vi "rs232_qsm.vi"   [LabVIEW 2013]
uses:
  labview/power_vi_stm_v13_1_7_22/labview/gen_libs/non_instr/gen_ctls/enums/state_enum.ctl
  labview/power_vi_stm_v13_1_7_22/labview/gen_libs/non_instr/gen_ctls/gen_ctls/ue_ref_clstr.ctl
  labview/power_vi_stm_v13_1_7_22/labview/gen_libs/instr/instr_ctls/instr_usr_evnt_clstr.ctl
  labview/power_vi_stm_v13_1_7_22/labview/gen_libs/instr/instr_ctls/res_tsk_out_clstr.ctl
  labview/power_vi_stm_v13_1_7_22/labview/gen_libs/instr/instr_ctls/keys_e36313a_params.ctl
  labview/power_vi_stm_v13_1_7_22/labview/projects/shell_to_shell/main_shell_to_shell_clstr.ctl
  labview/power_vi_stm_v13_1_7_22/labview/gen_libs/instr/instr_ctls/data_qtp_1133_clstr.ctl
  labview/power_vi_stm_v13_1_7_22/labview/gen_libs/instr/instr_ctls/ni_9205_params.ctl
  labview/power_vi_stm_v13_1_7_22/labview/gen_libs/instr/instr_ctls/ni_9213_params.ctl
  labview/power_vi_stm_v13_1_7_22/labview/gen_libs/instr/instr_ctls/ni_9205_volt_cal_params.ctl
  labview/power_vi_stm_v13_1_7_22/labview/gen_libs/both/gen_ctls/main_clstr.ctl
  labview/power_vi_stm_v13_1_7_22/labview/gen_libs/instr/instr_ctls/ni_8731a_params.ctl
  labview/power_vi_stm_v13_1_7_22/labview/gen_libs/non_instr/gen_ctls/gen_ctls/pwr_vi_test.ctl
  labview/power_vi_stm_v13_1_7_22/labview/gen_libs/instr/instr_ctls/ni_8731a_arry.ctl
  labview/power_vi_stm_v13_1_7_22/labview/gen_libs/instr/instr_ctls/dat_clstr_arry.ctl
  labview/power_vi_stm_v13_1_7_22/labview/gen_libs/instr/instr_ctls/watlow_std_bus.ctl
  labview/power_vi_stm_v13_1_7_22/labview/gen_libs/instr/instr_ctls/oven_settings.ctl
  labview/power_vi_stm_v13_1_7_22/labview/gen_libs/non_instr/gen_ctls/gen_ctls/gen_temp_cyc_clstr.ctl
  labview/power_vi_stm_v13_1_7_22/labview/gen_libs/instr/instr_ctls/daq_type_enum.ctl
  labview/power_vi_stm_v13_1_7_22/labview/gen_libs/instr/instr_ctls/source_type.ctl
  labview/power_vi_stm_v13_1_7_22/labview/gen_libs/instr/instr_ctls/daq_temp_enum.ctl
  labview/power_vi_stm_v13_1_7_22/labview/gen_libs/instr/instr_ctls/data_filtr_type_enum.ctl
  labview/power_vi_stm_v13_1_7_22/labview/gen_libs/instr/instr_ctls/when_to_soak_enum.ctl
  labview/power_vi_stm_v13_1_7_22/labview/gen_libs/instr/instr_ctls/tcp_rem_mon_enum.ctl
  labview/power_vi_stm_v13_1_7_22/labview/gen_libs/non_instr/gen_ctls/enums/temp_cond_enum.ctl
  labview/power_vi_stm_v13_1_7_22/labview/gen_libs/both/gen_ctls/rs232_data_clstr.ctl
  event_clstr.ctl
  states_cntrl.ctl
  log_dat.ctl
  temp_ind.ctl
  rh_ind_arry.ctl
  rh_ind.ctl
  sens_type.ctl
  sens_type_arry_cntrl.ctl
  pibs_clstr.ctl
  sens_type_arry_str_cntrl.ctl
  raw_dat_str.ctl
  dts_cntrl.ctl
types:
  T1 = typedef "rs232_data_clstr.ctl" = cluster{"state":T2, "connection ID":refnum<k5>, "stop_evnt_loop":bool, "main_q":refnum<queue>, "bytes read":u32, "Response":string, "wr_buffr":string, "bytes_at_port":u32, "visa_rsc_out":refnum<visa-resource-name>, "delay":u32, "sens_type_arry":T3, "chk_bytes_rd":u32}
  T2 = typedef "state_enum.ctl" = enum16{"idle", "exit", "obtain_q", "init", "create_file", "pik_sampl_mode", "init_instr_finite", "init_instr_cont", "update_file_path", "change_v_setting", "change _i_range", "turn_on_cur_qry", "turn_on_tst_cur", "dwell", "temp_stb_dwell", "meas", "v_set_qry", "range_qry", "save_data", "display_data", "cmd_proxy_state", "setting_proxy_state", "turn_off_tst_cur", "turn_off_curr_to_stop", "max_turn_off_trials_qry", "exit_prog", "max_trials_qry", "empty_str_qry", "man_cmd_qry", "man_cmd_qry_after_x_times", "cyc_qry", "turn_on_tcm", "turn_off_tcm", "chk_for_tcm", "max_trials_for_tcm", "turn_on_init_tcm", "srch_for_all_files", "strt_pdf_file", "append_pic", "append_header", "append_new_page", "pics_done_qry", "close_pdf_file", "set_cal_volt", "meas_cal_volt", "incr_voltage", "incr_cur_g1", "incr_cur_g2", "first_last_cyc_qry", "compare_results", "update_params", "cont_meas", "set_first_cur", "test_done_qry", "init_m3_temp_qry", "m3_diff_temp_qry", "temp_rched_qry", "set_init_oven_temp", "oven_temp_dwell", "update_oven_settings", "meas_oven_temp", "oven_temp_diff", "get_dat_from_vis", "ret_dat_from_cdaq", "ret_dat_from_ps", "close_cont_daqs", "cyc_trig_qry", "hot_temp_trig_qry", "cold_temp_trig_qry", "amb_temp_trig_qry", "both_temps_trig_qry", "temp_cond_hot_qry", "temp_cond_cold_qry", "temp_cond_amb_qry", "dur_strt_qry", "dur_end_qry", "daq_per_trig_qry", "src_type_qry", "turn_on_ps_1", "turn_off_ps_1", "turn_on_ps_2", "turn_off_ps_2", "data_type_qry", "user_stop_qry", "ret_data", "stm_snd_to_client", "strt_stm_listen", "snd_cmd", "capt_wait", "read_data", "chk_bytes_rd"}
  T3 = typedef "sens_type_arry_cntrl.ctl" = T4[]
  T4 = typedef "sens_type.ctl" = u8
  T5 = typedef "ue_ref_clstr.ctl" = cluster{"instr_usr_evnt_ref":refnum<user-event>, "key_e36313a_params_usr_evnt":refnum<user-event>, "main_stop_ue_ref":refnum<user-event>, "main_shell_to_shell_params":refnum<user-event>, "main_clstr_ref":refnum<user-event>, "stp_evnt_loop":refnum<user-event>}
  T6 = typedef "states_cntrl.ctl" = enum16{"idle", "exit", "init", "obtain_q", "capt_data", "snd_sens_type", "send_cmd", "capt_wait", "read_data", "chk_bytes_rd", "disp_data", "sav_qry", "sav_dat", "dwell", "small_dwell", "stop_capt_qry", "go_to_minor_qsm", "retr_data", "auto_in_minor_qsm"}
  T7 = typedef "event_clstr.ctl" = cluster{"states":T6, "bytes read":u32, "Response":string, "wr_buffr":string, "bytes_at_port":u32, "temp_clstr":T8, "logTable in":string[][][], "mult_list":i32, "log_tabl_row_cnt":u64, "above_row_7":bool, "sens_type":T4, "sens_type_arry":T3, "pibs_clstr":T12, "dts":T15}
  T8 = typedef "log_dat.ctl" = cluster{"sen_4_num":T9, "sen_3_num":T9, "sen_2_num":T9, "sen_1_num":T9, "sen_8_num":T9, "sen_7_num":T9, "sen_6_num":T9, "sen_5_num":T9, "dts":string, "sen_4":string, "sen_3":string, "sen_2":string, "sen_1":string, "sen_8":string, "sen_7":string, "sen_6":string, "sen_5":string, "temp_f_arry":T9[], "sens_dat_raw_arry":string[], "raw_dat":string, "rh_arry":T10, "rh_1":T11, "rh_0":T11, "rh_3":T11, "rh_2":T11, "rh_5":T11, "rh_4":T11, "rh_7":T11, "rh_6":T11}
  T9 = typedef "temp_ind.ctl" = dbl
  T10 = typedef "rh_ind_arry.ctl" = T11[]
  T11 = typedef "rh_ind.ctl" = dbl
  T12 = typedef "pibs_clstr.ctl" = cluster{"sens_typ_str":T13, "rh_1":T11, "sen_8":T14, "sen_7":T14, "sen_6":T14, "sen_5":T14, "sen_4":T14, "sen_3":T14, "sen_2":T14, "sen_1_num":T9, "sen_1":T14, "rh_2":T11, "rh_3":T11, "sen_2_num":T9, "sen_3_num":T9, "sen_4_num":T9, "rh_4":T11, "sen_5_num":T9, "rh_5":T11, "sen_6_num":T9, "rh_6":T11, "sen_7_num":T9, "rh_7":T11, "sen_8_num":T9, "rh_8":T11, "sens_type_1":T4, "sens_type_2":T4, "sens_type_3":T4, "sens_type_4":T4, "sens_type_5":T4, "sens_type_6":T4, "sens_type_7":T4, "sens_type_8":T4, "sens_typ_str _2":T13}
  T13 = typedef "sens_type_arry_str_cntrl.ctl" = string
  T14 = typedef "raw_dat_str.ctl" = string
  T15 = typedef "dts_cntrl.ctl" = string
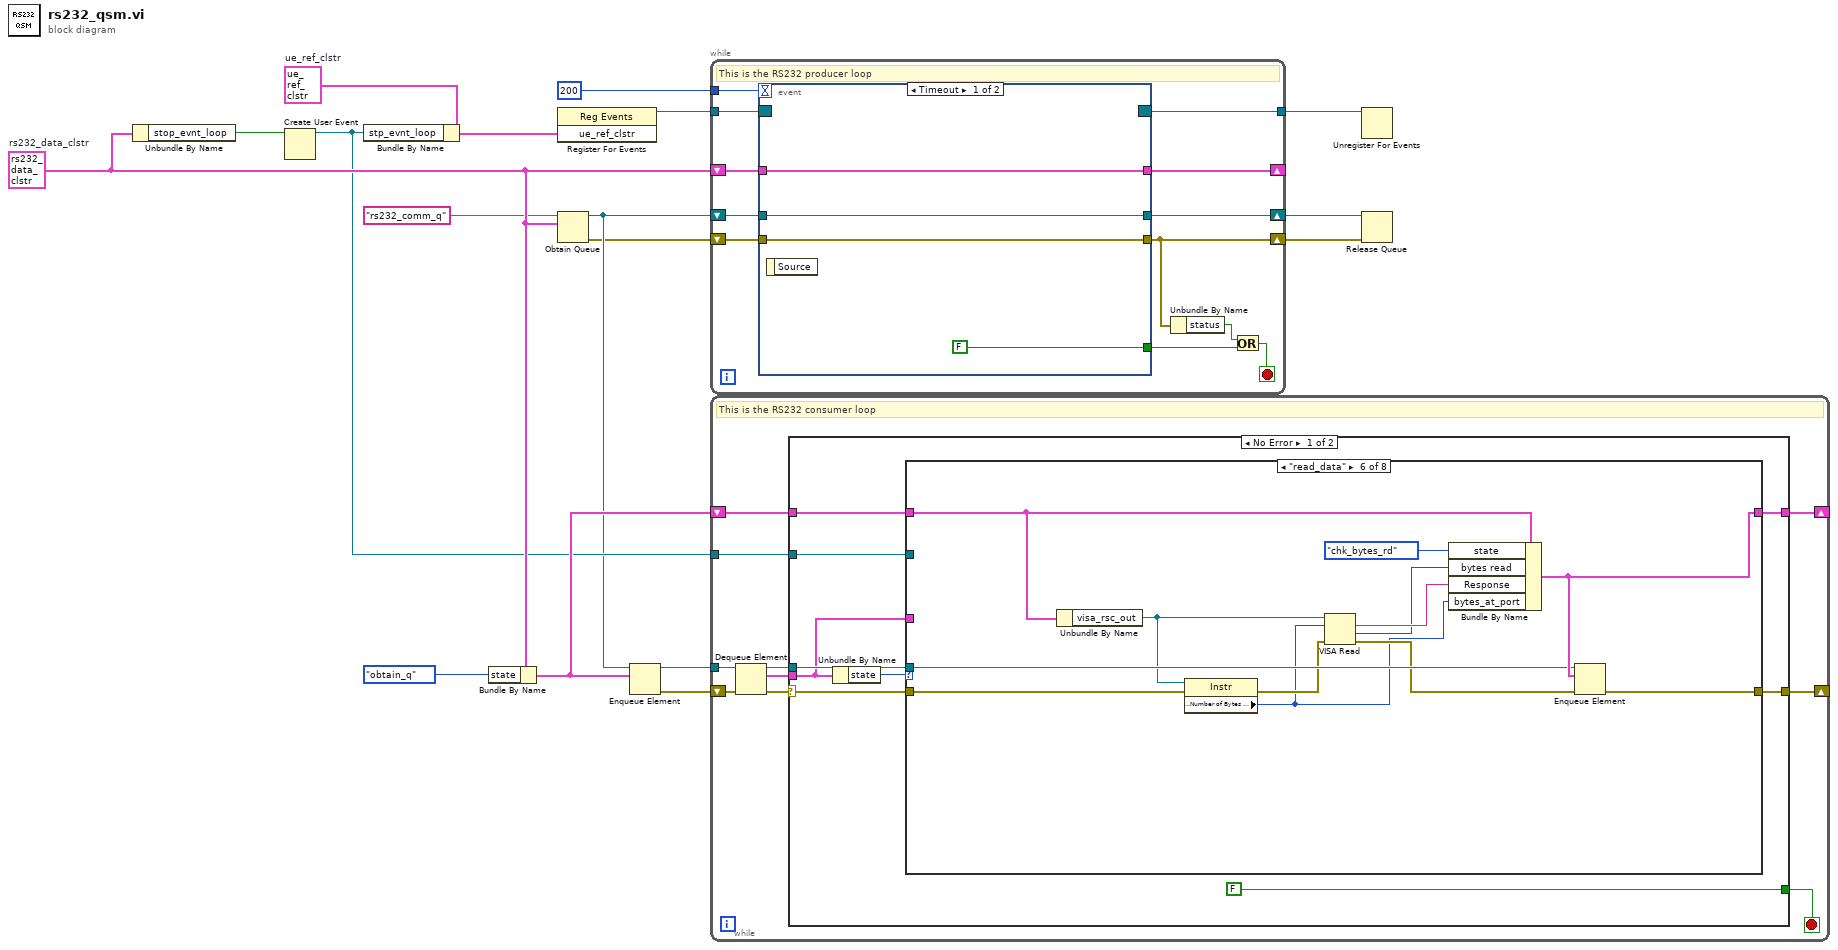
[diagram p0: block diagram]
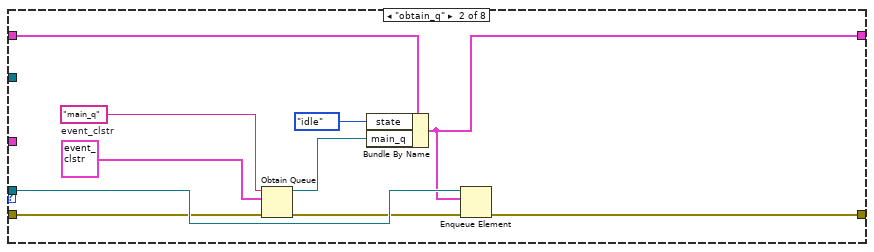
[diagram p3: hidden frame]
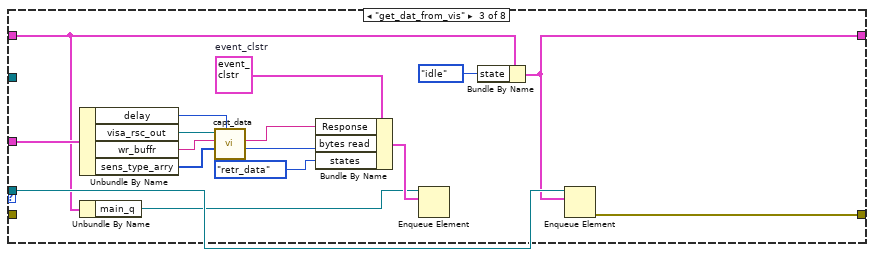
[diagram p4: hidden frame]
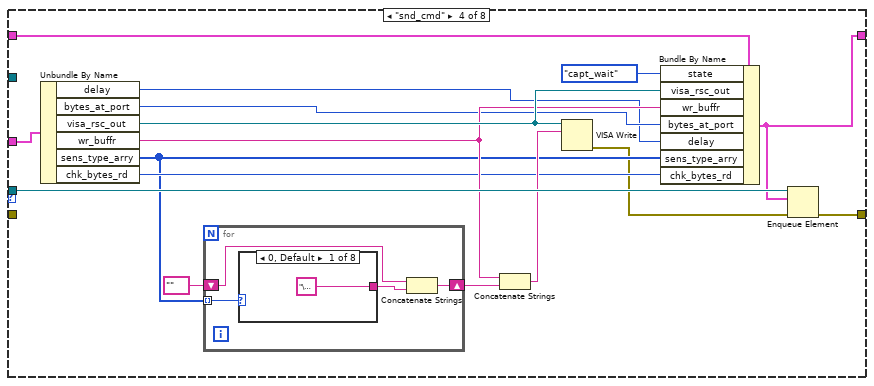
[diagram p5: hidden frame]
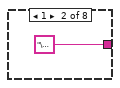
[diagram p6: hidden frame]
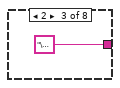
[diagram p7: hidden frame]
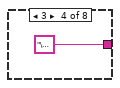
[diagram p8: hidden frame]
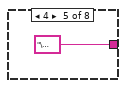
[diagram p9: hidden frame]
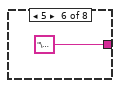
[diagram p10: hidden frame]
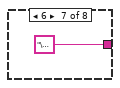
[diagram p11: hidden frame]
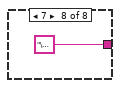
[diagram p12: hidden frame]
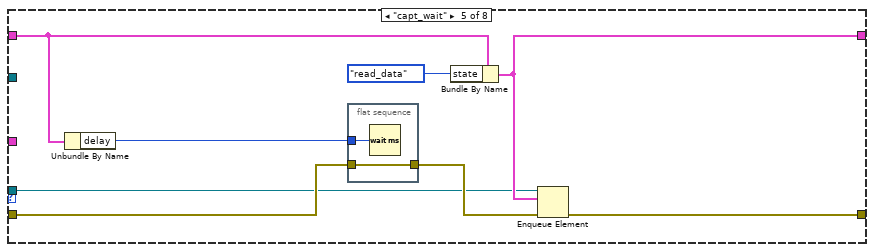
[diagram p13: hidden frame]
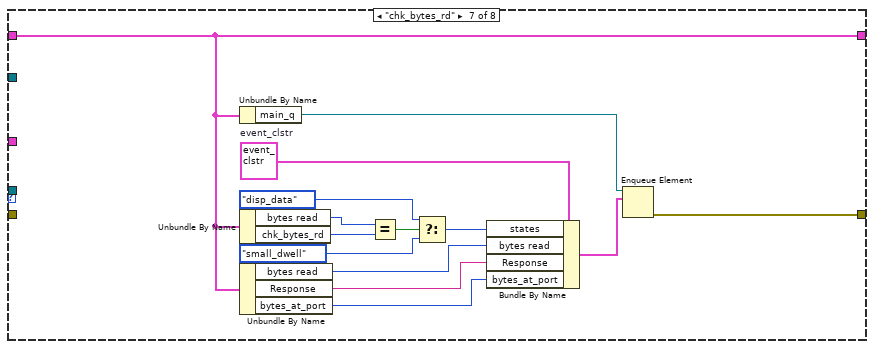
[diagram p14: hidden frame]
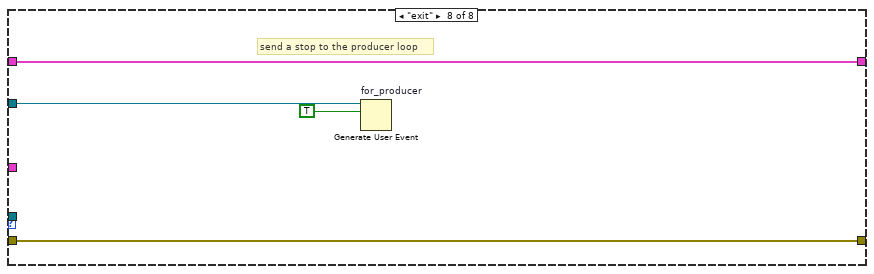
[diagram p15: hidden frame]
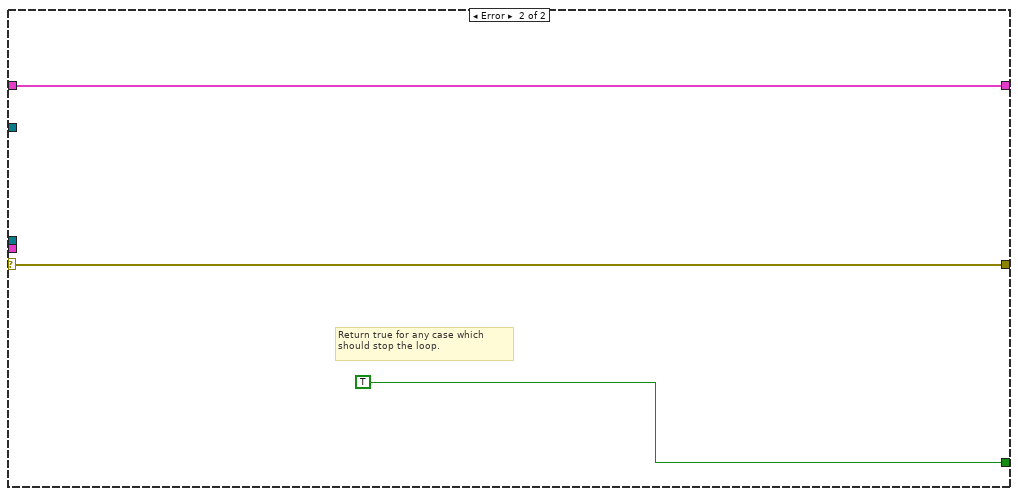
[diagram p16: hidden frame]
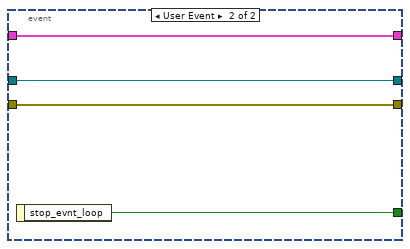
[diagram p17: hidden frame]
diagram:
  w17 = T1 {"state"=enum."idle", "connection ID"=refnum, "stop_evnt_loop"=FALSE, "main_q"=refnum, "bytes read"=0, "Response"="", "wr_buffr"="", "bytes_at_port"=0, "visa_rsc_out"="", "delay"=0, "sens_type_arry"=[], "chk_bytes_rd"=0}  # rs232_data_clstr
  w4 = T5 {"instr_usr_evnt_ref"=refnum, "key_e36313a_params_usr_evnt"=refnum, "main_stop_ue_ref"=refnum, "main_shell_to_shell_params"=refnum, "main_clstr_ref"=refnum, "stp_evnt_loop"=refnum}  # ue_ref_clstr
  n1 = Unbundle By Name(w17) -> ("stop_evnt_loop"=w5:bool)
  n2 = Create User Event(user event datatype=w5) -> (user event=w10:refnum<user-event>)  [unwired: 1 in, 1 out]
  n3 = Bundle By Name(cluster=w4, "stp_evnt_loop"=w10) -> (w3:T5)
  n4 = Bundle By Name(cluster=w17, "state"=state_enum."obtain_q") -> (w12:T1)
  n5 = register-events(w3) -> (reference out=w2:refnum<event-registration>)  [unwired: 2 in, 1 out]
  n6 = Obtain Queue(name (unnamed)="rs232_comm_q", element data type=w17) -> (queue out=w8:refnum<queue>, error out=w7:errorcluster)  [unwired: 3 in, 1 out]
  n7 = Enqueue Element(queue=w8, element=w12) -> (queue out=w9:refnum<queue>, error out=w13:errorcluster)  [unwired: 2 in, 1 out]
  n8 = while {
    shift-right: [w20] -> w16
    shift-left: w7 -> [w27]
    shift-right: [w28] -> w15
    shift-left: w8 -> [w29]
    shift-right: [w24] -> _
    shift-left: w17 -> [w26]
    tunnel: 200 -> [w25]
    tunnel: w2 -> [w23]
    tunnel: [w22] -> w14
    stop <- w18 stop-if-true
    # "This is the RS232 producer loop"
    n9 = event shown="[0] Timeout" {
      selector: w23 -> [_ _]
      dyn-events: [_ _] -> w22
      timeout: w25 -> [_ _]
      tunnel: w29 -> [w32 w36]
      tunnel: [w32 w36] -> w28
      tunnel: w27 -> [w31 w35]
      tunnel: [w31 w35] -> w20
      tunnel: w26 -> [w33 w37]
      tunnel: [w33 w37] -> w24
      tunnel: [FALSE w34] -> w19
      event Timeout {
        n10 = event-data() -> ()  [unwired: 1 in, 1 out]
      }
      event User Event {
        n11 = event-data() -> ("stop_evnt_loop"=w34:bool)  [unwired: 1 in]
      }
    }
    n12 = Unbundle By Name(w20) -> ("status"=w21:bool)
    n13 = Or(x=w21, y=w19) -> (x .or. y?=w18:bool)
  }
  n14 = while {
    tunnel: w9 -> [w47]
    shift-right: [w42] -> _
    shift-left: w12 -> [w43]
    shift-right: [w40] -> _
    shift-left: w13 -> [w44]
    tunnel: w10 -> [w39]
    stop <- w38 stop-if-true
    # "This is the RS232 consumer loop"
    n15 = Dequeue Element(queue=w47, error in (no error)=w44) -> (queue out=w41:refnum<queue>, element=w45:T1, error out=w46:errorcluster)  [unwired: 1 in, 1 out]
    n16 = case shown="No Error" w46 {
      selector: w46 -> [w55 w153]
      tunnel: w45 -> [w49 _]
      tunnel: [FALSE TRUE] -> w38
      tunnel: w43 -> [w54 w154]
      tunnel: [w48 w154] -> w42
      tunnel: w41 -> [w53 _]
      tunnel: [w52 w153] -> w40
      tunnel: w39 -> [w50 _]
      frame No Error {
        n17 = Unbundle By Name(w49) -> ("state"=w56:T2)
        n18 = case shown="\"read_data\"" w56 {
          tunnel: w55 -> [w58 w65 _ _ w116 w129 _ w152]
          tunnel: w54 -> [w57 w62 w71 w97 w113 w124 w138 w149]
          tunnel: w53 -> [_ w67 w72 w98 w114 w131 _ _]
          tunnel: [w58 w66 w83 w99 w119 w133 w148 w152] -> w52
          tunnel: w50 -> [_ _ _ _ _ _ _ w151]
          tunnel: w49 -> [_ _ w78 w93 _ _ _ _]
          tunnel: [w57 w59 w69 w96 w118 w132 w138 w149] -> w48
          frame "idle", Default {
          }
          frame "obtain_q" {
            w61 = T7 {"states"=enum."init", "bytes read"=7, "Response"="á7Mìhc\u000b", "wr_buffr"="\b", "bytes_at_port"=0, "temp_clstr"={"sen_4_num"=0.0, "sen_3_num"=0.0, "sen_2_num"=0.0, "sen_1_num"=0.0, "sen_8_num"=0.0, "sen_7_num"=0.0, "sen_6_num"=0.0, "sen_5_num"=0.0, "dts"="", "sen_4"="", "sen_3"="", "sen_2"="", "sen_1"="", "sen_8"="", "sen_7"="", "sen_6"="", "sen_5"="", "temp_f_arry"=[], "sens_dat_raw_arry"=[], "raw_dat"="", "rh_arry"=[], "rh_1"=0.0, "rh_0"=0.0, "rh_3"=0.0, "rh_2"=0.0, "rh_5"=0.0, "rh_4"=0.0, "rh_7"=0.0, "rh_6"=0.0}, "logTable in"=[], "mult_list"=0, "log_tabl_row_cnt"=0, "above_row_7"=FALSE, "sens_type"=0, "sens_type_arry"=[], "pibs_clstr"={"sens_typ_str"="", "rh_1"=0.0, "sen_8"="", "sen_7"="", "sen_6"="", "sen_5"="", "sen_4"="", "sen_3"="", "sen_2"="", "sen_1_num"=0.0, "sen_1"="", "rh_2"=0.0, "rh_3"=0.0, "sen_2_num"=0.0, "sen_3_num"=0.0, "sen_4_num"=0.0, "rh_4"=0.0, "sen_5_num"=0.0, "rh_5"=0.0, "sen_6_num"=0.0, "rh_6"=0.0, "sen_7_num"=0.0, "rh_7"=0.0, "sen_8_num"=0.0, "rh_8"=0.0, "sens_type_1"=0, "sens_type_2"=0, "sens_type_3"=0, "sens_type_4"=0, "sens_type_5"=0, "sens_type_6"=0, "sens_type_7"=0, "sens_type_8"=0, "sens_typ_str _2"=""}, "dts"=""}  # event_clstr
            n19 = Obtain Queue(name (unnamed)="main_q", element data type=w61, error in (no error)=w65) -> (queue out=w60:refnum<queue>, error out=w64:errorcluster)  [unwired: 2 in, 1 out]
            n20 = Bundle By Name(cluster=w62, "state"=state_enum."idle", "main_q"=w60) -> (w59:T1)
            n21 = Enqueue Element(queue=w67, element=w59, error in (no error)=w64) -> (error out=w66:errorcluster)  [unwired: 1 in, 2 out]
          }
          frame "get_dat_from_vis" {
            w74 = T7 {"states"=enum."idle", "bytes read"=0, "Response"="", "wr_buffr"="\b", "bytes_at_port"=0, "temp_clstr"={"sen_4_num"=0.0, "sen_3_num"=0.0, "sen_2_num"=0.0, "sen_1_num"=0.0, "sen_8_num"=0.0, "sen_7_num"=0.0, "sen_6_num"=0.0, "sen_5_num"=0.0, "dts"="", "sen_4"="", "sen_3"="", "sen_2"="", "sen_1"="", "sen_8"="", "sen_7"="", "sen_6"="", "sen_5"="", "temp_f_arry"=[], "sens_dat_raw_arry"=[], "raw_dat"="", "rh_arry"=[], "rh_1"=0.0, "rh_0"=0.0, "rh_3"=0.0, "rh_2"=0.0, "rh_5"=0.0, "rh_4"=0.0, "rh_7"=0.0, "rh_6"=0.0}, "logTable in"=[], "mult_list"=0, "log_tabl_row_cnt"=0, "above_row_7"=FALSE, "sens_type"=0, "sens_type_arry"=[], "pibs_clstr"={"sens_typ_str"="", "rh_1"=0.0, "sen_8"="", "sen_7"="", "sen_6"="", "sen_5"="", "sen_4"="", "sen_3"="", "sen_2"="", "sen_1_num"=0.0, "sen_1"="", "rh_2"=0.0, "rh_3"=0.0, "sen_2_num"=0.0, "sen_3_num"=0.0, "sen_4_num"=0.0, "rh_4"=0.0, "sen_5_num"=0.0, "rh_5"=0.0, "sen_6_num"=0.0, "rh_6"=0.0, "sen_7_num"=0.0, "rh_7"=0.0, "sen_8_num"=0.0, "rh_8"=0.0, "sens_type_1"=0, "sens_type_2"=0, "sens_type_3"=0, "sens_type_4"=0, "sens_type_5"=0, "sens_type_6"=0, "sens_type_7"=0, "sens_type_8"=0, "sens_typ_str _2"=""}, "dts"=""}  # event_clstr
            n22 = Unbundle By Name(w78) -> ("delay"=w80:u32, "visa_rsc_out"=w82:refnum<visa-resource-name>, "wr_buffr"=w81:string, "sens_type_arry"=w79:T3)
            n23 = Unbundle By Name(w71) -> ("main_q"=w70:refnum<queue>)
            n24 = call "capt_data.vi"("delay before read (ms)"=w80, "sens_type_arry"=w79, "wr_buffr"=w81, "VISA Refnum in"=w82) -> ("bytes read"=w76:u32, "Response"=w77:string)  [unwired: 4 in, 2 out]
            n25 = Bundle By Name(cluster=w74, "Response"=w77, "bytes read"=w76, "states"=states_cntrl."retr_data") -> (w75:T7)
            n26 = Enqueue Element(queue=w70, element=w75) -> ()  [unwired: 2 in, 3 out]
            n27 = Bundle By Name(cluster=w71, "state"=state_enum."idle") -> (w69:T1)
            n28 = Enqueue Element(queue=w72, element=w69) -> (error out=w83:errorcluster)  [unwired: 2 in, 2 out]
          }
          frame "snd_cmd" {
            n29 = Unbundle By Name(w93) -> ("delay"=w86:u32, "bytes_at_port"=w89:u32, "visa_rsc_out"=w91:refnum<visa-resource-name>, "wr_buffr"=w90:string, "sens_type_arry"=w87:T3, "chk_bytes_rd"=w88:u32)
            n30 = for {
              tunnel: w87 -> [w103] mode=indexing
              shift-right: [w102] -> w95
              shift-left: "" -> [w104]
              n31 = case shown="0, Default" w103 {
                tunnel: ["\u0000" "\u0001" "\u0002" "\u0003" "\u0004" "\u0005" "\u0006" "\u0007"] -> w101
                frame 0, Default {
                }
                frame 1 {
                }
                frame 2 {
                }
                frame 3 {
                }
                frame 4 {
                }
                frame 5 {
                }
                frame 6 {
                }
                frame 7 {
                }
              }
              n32 = Concatenate Strings(w104, w101) -> (w102:string)
            }
            n33 = Concatenate Strings(w90, w95) -> (w92:string)
            n34 = VISA Write(VISA resource name=w91, write buffer=w92) -> (error out=w85:errorcluster)  [unwired: 1 in, 2 out]
            n35 = Bundle By Name(cluster=w97, "state"=state_enum."capt_wait", "visa_rsc_out"=w91, "wr_buffr"=w90, "bytes_at_port"=w89, "delay"=w86, "sens_type_arry"=w87, "chk_bytes_rd"=w88) -> (w96:T1)
            n36 = Enqueue Element(queue=w98, element=w96, error in (no error)=w85) -> (error out=w99:errorcluster)  [unwired: 1 in, 2 out]
          }
          frame "capt_wait" {
            n37 = Unbundle By Name(w113) -> ("delay"=w117:u32)
            n38 = flat-sequence {
              tunnel: w117 -> [w122]
              tunnel: [w121] -> w115
              tunnel: w116 -> [w121]
              frame #0 {
                n39 = Wait (ms)(milliseconds to wait=w122) -> ()  [unwired: 1 out]
              }
            }
            n40 = Bundle By Name(cluster=w113, "state"=state_enum."read_data") -> (w118:T1)
            n41 = Enqueue Element(queue=w114, element=w118, error in (no error)=w115) -> (error out=w119:errorcluster)  [unwired: 1 in, 2 out]
          }
          frame "read_data" {
            n42 = Unbundle By Name(w124) -> ("visa_rsc_out"=w123:refnum<visa-resource-name>)
            n43 = property class="Instr"(reference=w123, error in=w129) -> (error out=w130:errorcluster, "Serial Settings:Number of Bytes at Serial Port"=w126:u32)  [unwired: 1 out]
            n44 = VISA Read(VISA resource name=w123, byte count=w126, error in (no error)=w130) -> (read buffer=w127:string, return count=w125:u32, error out=w128:errorcluster)  [unwired: 1 out]
            n45 = Bundle By Name(cluster=w124, "state"=state_enum."chk_bytes_rd", "bytes read"=w125, "Response"=w127, "bytes_at_port"=w126) -> (w132:T1)
            n46 = Enqueue Element(queue=w131, element=w132, error in (no error)=w128) -> (error out=w133:errorcluster)  [unwired: 1 in, 2 out]
          }
          frame "chk_bytes_rd" {
            w141 = T7 {"states"=enum."idle", "bytes read"=0, "Response"="", "wr_buffr"="\b", "bytes_at_port"=0, "temp_clstr"={"sen_4_num"=0.0, "sen_3_num"=0.0, "sen_2_num"=0.0, "sen_1_num"=0.0, "sen_8_num"=0.0, "sen_7_num"=0.0, "sen_6_num"=0.0, "sen_5_num"=0.0, "dts"="", "sen_4"="", "sen_3"="", "sen_2"="", "sen_1"="", "sen_8"="", "sen_7"="", "sen_6"="", "sen_5"="", "temp_f_arry"=[], "sens_dat_raw_arry"=[], "raw_dat"="", "rh_arry"=[], "rh_1"=0.0, "rh_0"=0.0, "rh_3"=0.0, "rh_2"=0.0, "rh_5"=0.0, "rh_4"=0.0, "rh_7"=0.0, "rh_6"=0.0}, "logTable in"=[], "mult_list"=0, "log_tabl_row_cnt"=0, "above_row_7"=FALSE, "sens_type"=0, "sens_type_arry"=[], "pibs_clstr"={"sens_typ_str"="", "rh_1"=0.0, "sen_8"="", "sen_7"="", "sen_6"="", "sen_5"="", "sen_4"="", "sen_3"="", "sen_2"="", "sen_1_num"=0.0, "sen_1"="", "rh_2"=0.0, "rh_3"=0.0, "sen_2_num"=0.0, "sen_3_num"=0.0, "sen_4_num"=0.0, "rh_4"=0.0, "sen_5_num"=0.0, "rh_5"=0.0, "sen_6_num"=0.0, "rh_6"=0.0, "sen_7_num"=0.0, "rh_7"=0.0, "sen_8_num"=0.0, "rh_8"=0.0, "sens_type_1"=0, "sens_type_2"=0, "sens_type_3"=0, "sens_type_4"=0, "sens_type_5"=0, "sens_type_6"=0, "sens_type_7"=0, "sens_type_8"=0, "sens_typ_str _2"=""}, "dts"=""}  # event_clstr
            n47 = Unbundle By Name(w138) -> ("main_q"=w142:refnum<queue>)
            n48 = Unbundle By Name(w138) -> ("bytes read"=w144:u32, "chk_bytes_rd"=w143:u32)
            n49 = Unbundle By Name(w138) -> ("bytes read"=w137:u32, "Response"=w136:string, "bytes_at_port"=w135:u32)
            n50 = Equal?(x=w144, y=w143) -> (x = y?=w145:bool)
            n51 = Select(t=states_cntrl."disp_data" ("states"), s=w145, f=states_cntrl."small_dwell") -> (s? t:f=w140:T6)
            n52 = Bundle By Name(cluster=w141, "states"=w140, "bytes read"=w137, "Response"=w136, "bytes_at_port"=w135) -> (w139:T7)
            n53 = Enqueue Element(queue=w142, element=w139) -> (error out=w148:errorcluster)  [unwired: 2 in, 2 out]
          }
          frame "exit" {
            # "send a stop to the producer loop"
            n54 = Generate User Event "for_producer"(user event=w151, event data cluster=TRUE) -> ()  [unwired: 2 in, 2 out]
          }
        }
      }
      frame Error {
        # "Return true for any case which should stop the loop."
      }
    }
  }
  n55 = Unregister For Events(event registration refnum=w14) -> ()  [unwired: 1 in, 1 out]
  n56 = Release Queue(queue=w15, error in (no error)=w16) -> ()  [unwired: 1 in, 3 out]
